vi "Build Array of References.vi"(6 "Variant in":variant, 7 "Shift Pressed?":bool, 8 "error in (no error)":errorcluster, 10 "QD Combo Box Ref":refnum<vi>, 11 "QD Launch VI Ref":refnum<vi>) -> (0 "error out":errorcluster, 4 "Variant out":variant)   [LabVIEW 2020]
doc: "### Build Array of Reference/Build Cluster of Reference\n\nCreate references with 'Build Array'/'buddle' together.\n\nDefault Shortcut - [B]"
uses:
  _support/Build Array of References__RCF.lvlib
panel:
  in  "Undo Name":string="Quick Drop Keyboard Shortcut"
  # "Do not change the connector pane of this VI.\n\nSee the block diagram for directions on how to use this template."
  # "Specify the name of the Undo transaction"
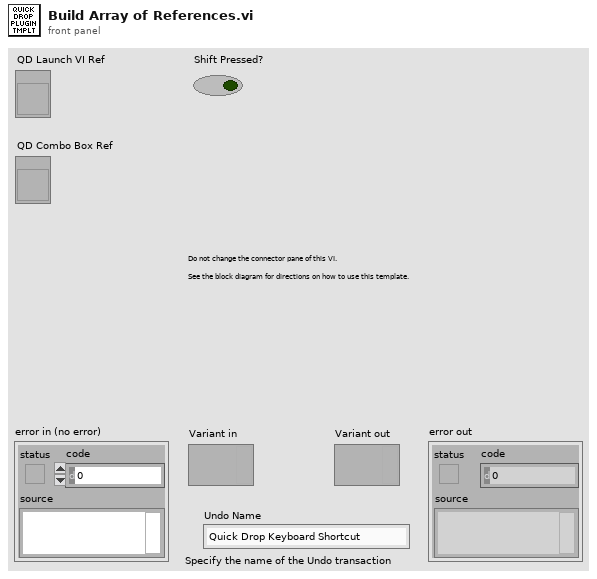
[diagram p1: front panel]
types:
  T1 = cluster{"ItemTag":string, "ItemPath":string, "Coords":cluster{"Horizontal":i32, "Vertical":i32}}
  T2 = cluster{"Active VI Refnum":refnum<vi>, "Active VI Type":enum16{"Panel", "Diagram"}, "Active VI Sel. List[]":refnum<vi>[], "Mouse Coords":cluster{"Horizontal":i32, "Vertical":i32}}
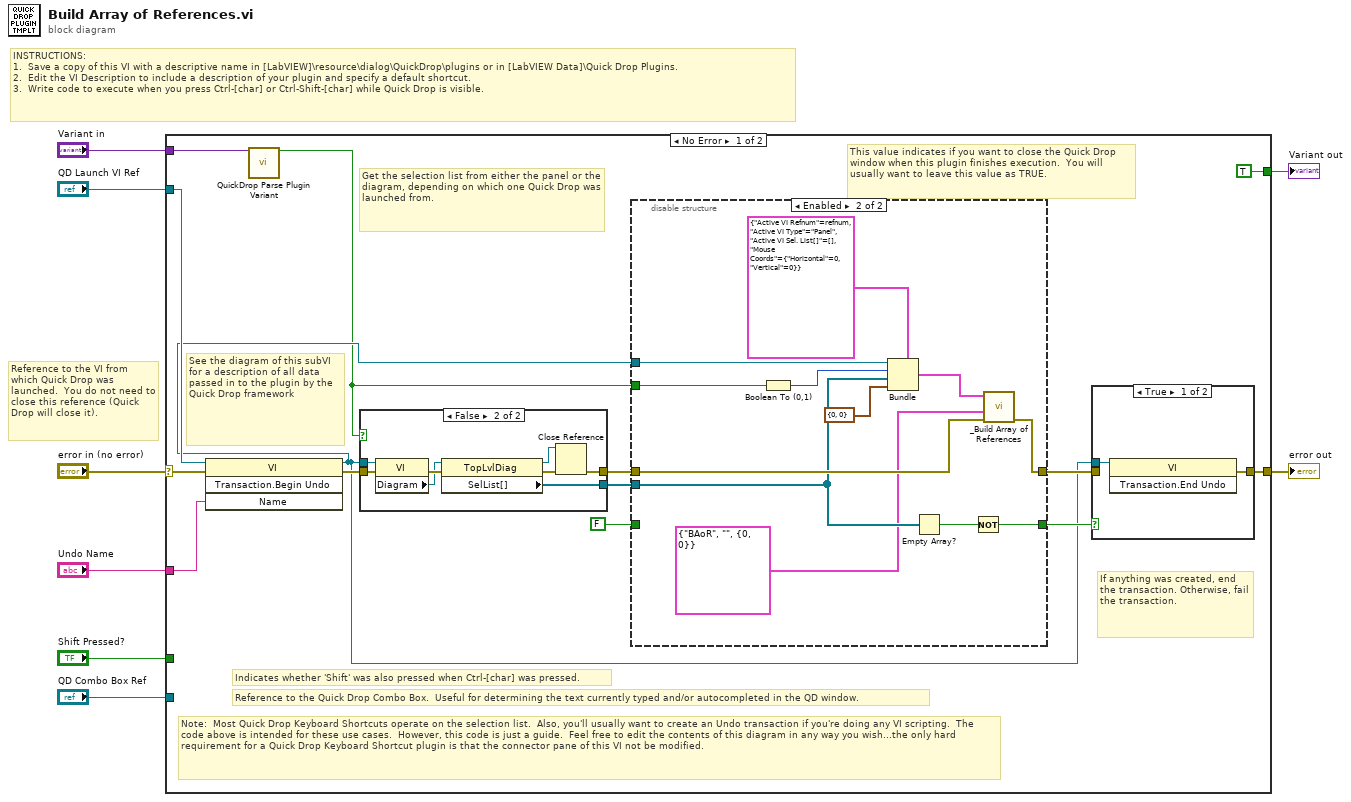
[diagram p0: block diagram]
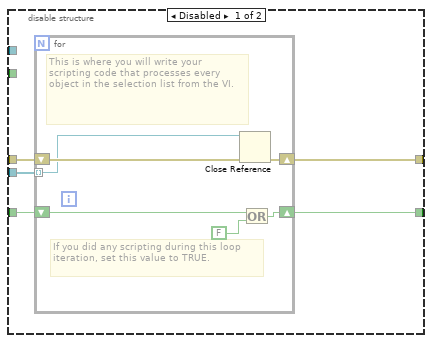
[diagram p2: hidden frame]
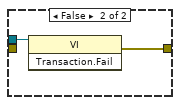
[diagram p3: hidden frame]
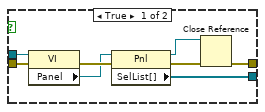
[diagram p4: hidden frame]
diagram:
  # "Reference to the VI from which Quick Drop was launched.  You do not need to close this reference (Quick Drop will close it)."
  # "INSTRUCTIONS:\n1.  Save a copy of this VI with a descriptive name in [LabVIEW]\\resource\\dialog\\QuickDrop\\plugins or in [LabVIEW Data]\\Quick Drop Plugins.\n2.  Edit the VI Description to include a description of your plugin and specify a default shortcut. \n3.  Write code to execute when you press Ctrl-[char] or Ctrl-Shift-[char] while Quick Drop is visible."
  n1 = case shown="No Error" "error in (no error)" {
    selector: "error in (no error)" -> [w21 w66]
    tunnel: [w16 w66] -> w7
    tunnel: "QD Launch VI Ref" -> [w20 _]
    tunnel: "Shift Pressed?" -> [_ _]
    tunnel: "QD Combo Box Ref" -> [_ _]
    tunnel: "Variant in" -> [w22 _]
    tunnel: "Undo Name" -> [w19 _]
    tunnel: [TRUE _] -> w1
    frame No Error {
      # "Note:  Most Quick Drop Keyboard Shortcuts operate on the selection list.  Also, you'll usually want to create an Undo transaction if you're doing any VI scripting.  The code above is intended for these use cases.  However, this code is just a guide.  Feel free to edit the contents of this diagram in any way you wish...the only hard requirement for a Quick Drop Keyboard Shortcut plugin is that the connector pane of this VI not be modified."
      # "Get the selection list from either the panel or the diagram, depending on which one Quick Drop was launched from."
      # "If anything was created, end the transaction. Otherwise, fail the transaction."
      # "This value indicates if you want to close the Quick Drop window when this plugin finishes execution.  You will usually want to leave this value as TRUE."
      # "See the diagram of this subVI for a description of all data passed in to the plugin by the Quick Drop framework"
      # "Reference to the Quick Drop Combo Box.  Useful for determining the text currently typed and/or autocompleted in the QD window."
      # "Indicates whether 'Shift' was also pressed when Ctrl-[char] was pressed."
      n2 = invoke class="VI" method="Transaction.Begin Undo"(reference=w20, error in=w21, "Name"=w19) -> (reference out=w10:refnum<vi>, error out=w17:errorcluster)  [unwired: 1 in, 2 out]
      n3 = call <vilib>:"QuickDrop Parse Plugin Variant.vi"("QDKS Variant in"=w22) -> ("QD Launch VI Panel?"=w9:bool)  [unwired: 12 in, 2 out]
      n4 = case shown="False" w9 {
        tunnel: w17 -> [w57 w65]
        tunnel: w10 -> [w56 w64]
        tunnel: [w51 w59] -> w15
        tunnel: [w50 w58] -> w11
        frame True {
          n5 = property class="VI"(reference=w56, error in=w57) -> (error out=w55:errorcluster, "Panel"=w54:refnum<vi>)  [unwired: 1 out]
          n6 = property class="Pnl"(reference=w54, error in=w55) -> (reference out=w52:refnum<vi>, error out=w53:errorcluster, "SelList[]"=w50:refnum<vi>[])
          n7 = Close Reference(reference=w52, error in (no error)=w53) -> (error out=w51:errorcluster)
        }
        frame False {
          n8 = property class="VI"(reference=w64, error in=w65) -> (error out=w63:errorcluster, "Diagram"=w62:refnum<vi>)  [unwired: 1 out]
          n9 = property class="TopLvlDiag"(reference=w62, error in=w63) -> (reference out=w60:refnum<vi>, error out=w61:errorcluster, "SelList[]"=w58:refnum<vi>[])
          n10 = Close Reference(reference=w60, error in (no error)=w61) -> (error out=w59:errorcluster)
        }
      }
      n11 = disable-structure shown="Enabled" {
        disable-tunnel: w15 -> [w27 w39]
        disable-tunnel: [w26 w38] -> w14
        disable-tunnel: FALSE -> [w25 _]
        disable-tunnel: [w24 w35] -> w12
        disable-tunnel: w11 -> [w23 w36]
        disable-tunnel: w10 -> [_ w44]
        disable-tunnel: w9 -> [_ w43]
        frame Disabled {
          n12 = for {
            shift-right: [w29] -> w26
            shift-left: w27 -> [w30]
            shift-right: [w32] -> w24
            shift-left: w25 -> [w33]
            tunnel: w23 -> [w28] mode=indexing
            # "This is where you will write your scripting code that processes every object in the selection list from the VI."
            # "If you did any scripting during this loop iteration, set this value to TRUE."
            n13 = Close Reference(reference=w28, error in (no error)=w30) -> (error out=w29:errorcluster)
            n14 = Or(x=w33, y=FALSE ("x")) -> (x .or. y?=w32:bool)
          }
        }
        frame Enabled {
          n15 = Boolean To (0,1)(Boolean=w43) -> (0, 1=w42:i16)
          n16 = Bundle(cluster=T2 {"Active VI Refnum"=refnum, "Active VI Type"=enum."Panel", "Active VI Sel. List[]"=[], "Mouse Coords"={"Horizontal"=0, "Vertical"=0}} ("Active VI Info"), "Active VI Refnum"=w44, "Active VI Type"=w42, "Active VI Sel. List[]"=w36, "Mouse Coords"=cluster{"Horizontal":i32, "Vertical":i32} {"Horizontal"=0, "Vertical"=0}) -> (w40:T2)
          n17 = Empty Array?(array=w36) -> (empty?=w37:bool)
          n18 = Not(x=w37) -> (.not. x?=w35:bool)
          n19 = call "_Build Array of References.vi"("error in"=w39, "Shortcut Menu Selection"=T1 {"ItemTag"="BAoR", "ItemPath"="", "Coords"={"Horizontal"=0, "Vertical"=0}}, "Active VI Info"=w40) -> ("error out"=w38:errorcluster)  [unwired: 8 in]
        }
      }
      n20 = case shown="True" w12 {
        tunnel: w10 -> [w46 w48]
        tunnel: [w47 w49] -> w16
        tunnel: w14 -> [_ _]
        frame True {
          n21 = invoke class="VI" method="Transaction.End Undo"(reference=w46) -> (error out=w47:errorcluster)  [unwired: 2 in, 2 out]
        }
        frame False {
          n22 = invoke class="VI" method="Transaction.Fail"(reference=w48) -> (error out=w49:errorcluster)  [unwired: 2 in, 2 out]
        }
      }
    }
    frame Error {
    }
  }
  "error out" <- w7
  "Variant out" <- w1
